vi "changeDigitalFilter.vi"(8 "error in (no error)":errorcluster, 10 "ElectrometerController in":refnum<class "ElectrometerController.lvclass">, 11 "State in":refnum<class "ReadyState.lvclass">) -> (0 "error out":errorcluster, 2 "ElectrometerController out":refnum<class "ElectrometerController.lvclass">, 3 "State out":refnum<class "ReadyState.lvclass">)   [LabVIEW 2016, in "ReadyState.lvclass"]
uses:
  ReadyState.lvclass
  ElectrometerController/ElectrometerController.lvclass
  internalState.ctl
  Electrometer.lvclass
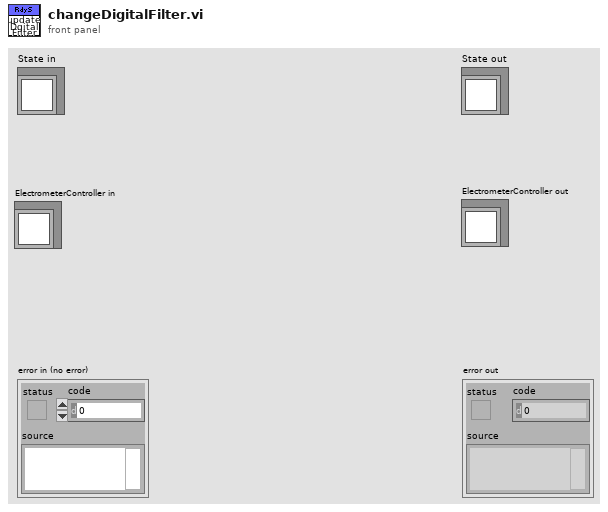
[diagram p1: front panel]
types:
  T1 = typedef "Electrometer.lvclass/internalState.ctl" = enum16{"Ready", "Configuring", "ManualReading", "UntilIntensityReading", "SetDurationReading", "BufferReading"}
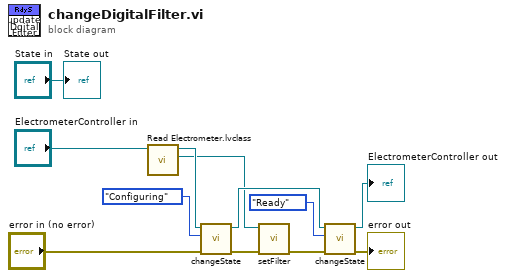
[diagram p0: block diagram]
diagram:
  n1 = call-dynamic "Read Electrometer.lvclass.vi"("ElectrometerController in"="ElectrometerController in") -> ("Electrometer.lvclass"=w3:refnum<class "Electrometer.lvclass">, "ElectrometerController out"=w11:refnum<class "ElectrometerController.lvclass">)  [unwired: 8 in, 1 out]
  n2 = call "changeState.vi"("error in (no error)"="error in (no error)", "State"=internalState."Configuring" ("States"), "ElectrometerController in"=w11) -> ("error out"=w2:errorcluster, "ElectrometerController out"=w9:refnum<class "ElectrometerController.lvclass">)  [unwired: 7 in]
  n3 = call "setFilter.vi"("error in (no error)"=w2, "Electrometer in"=w3) -> ("error out"=w1:errorcluster)  [unwired: 8 in, 1 out]
  n4 = call "changeState.vi"("error in (no error)"=w1, "State"=internalState."Ready" ("States"), "ElectrometerController in"=w9) -> ("error out"=→"error out":errorcluster, "ElectrometerController out"=→"ElectrometerController out":refnum<class "ElectrometerController.lvclass">)  [unwired: 7 in]
  "State out" <- "State in"
